vi "tm_getdcimgframes16_40.vi"(7 "Options":i32(ring) items=["no option"=0, "high contrast"=16], 8 "error in (no error)":errorcluster, 10 "Frame Index":i32=-1, 11 "File Handle in":u32) -> (0 "error out":errorcluster, 1 "Data B":u16[][](array[numeric]), 2 "Data A":u16[][](array[numeric]), 3 "File Handle out":u32, 4 "Timestamp":dbl)   [LabVIEW 2023]
uses:
  tmcamcon.dll
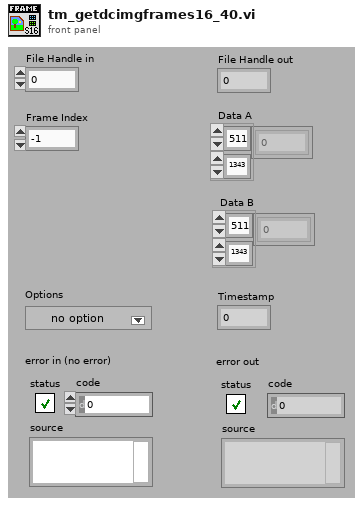
[diagram p1: front panel]
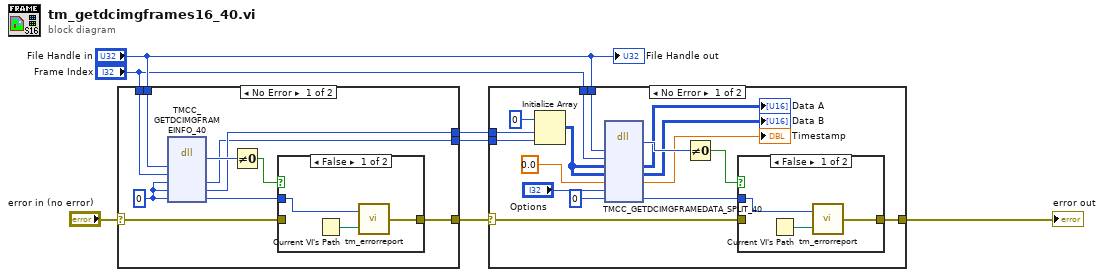
[diagram p0: block diagram]
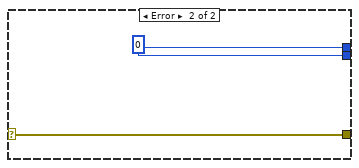
[diagram p5: hidden frame]
diagram:
  n1 = case shown="No Error" "error in (no error)" {
    selector: "error in (no error)" -> [w11 w23]
    tunnel: [w8 w23] -> w6
    tunnel: "File Handle in" -> [w16 _]
    tunnel: [w12 w22] -> w3
    tunnel: [w13 w22] -> w4
    tunnel: "Frame Index" -> [w14 _]
    frame No Error {
      w15 = 0 ("Erval")
      n2 = dll-call lib="tmcamcon.dll" fn="TMCC_GETDCIMGFRAMEINFO_40"("index"=w16, "frameindex"=w14, "width"=w15, "height"=w15, "Erval"=w15) -> ("return type"=w17:u32, "width"=w12:i32, "height"=w13:i32, "Erval"=w10:i32)  [unwired: 5 in, 2 out]
      n3 = Not Equal To 0?(x=w17) -> (x != 0?=w9:bool)
      n4 = case shown="False" w9 {
        tunnel: w11 -> [_ w21]
        tunnel: [w19 w21] -> w8
        tunnel: w10 -> [w18 _]
        frame False {
          n5 = Current VI's Path() -> (path=w20:path)
          n6 = call "tm_errorreport.vi"("Source"=w20, "Error"=w18) -> ("error out"=w19:errorcluster)
        }
        frame True {
        }
      }
    }
    frame Error {
      w22 = 0 ("buf")
    }
  }
  n7 = case shown="No Error" w6 {
    selector: w6 -> [w30 w45]
    tunnel: [w27 w45] -> w2
    tunnel: "File Handle in" -> [w39 _]
    tunnel: w4 -> [w37 _]
    tunnel: w3 -> [w36 _]
    tunnel: "Frame Index" -> [w34 _]
    frame No Error {
      n8 = Initialize Array(u16 0 ("buf"), w37, w36) -> (w25:u16[][])
      n9 = dll-call lib="tmcamcon.dll" fn="TMCC_GETDCIMGFRAMEDATA_SPLIT_40"("index"=w39, "frame"=w34, "imgarray1"=w25, "imgarray2"=w25, "timestamp"=0.0 ("Erval"), "option"="Options", "Erval"=0) -> ("return type"=w40:u32, "imgarray1"=→"Data A":u16[][], "imgarray2"=→"Data B":u16[][], "timestamp"=→"Timestamp":dbl, "Erval"=w29:i32)  [unwired: 6 in, 2 out]
      n10 = Not Equal To 0?(x=w40) -> (x != 0?=w28:bool)
      n11 = case shown="False" w28 {
        tunnel: w30 -> [_ w44]
        tunnel: [w42 w44] -> w27
        tunnel: w29 -> [w41 _]
        frame False {
          n12 = Current VI's Path() -> (path=w43:path)
          n13 = call "tm_errorreport.vi"("Source"=w43, "Error"=w41) -> ("error out"=w42:errorcluster)
        }
        frame True {
        }
      }
    }
    frame Error {
    }
  }
  "error out" <- w2
  "File Handle out" <- "File Handle in"
